vi "Make All Characters Displayable.vi"(11 "String In":string) -> (3 "Escaped String":string)   [LabVIEW 2015, in "VITAC.lvlib"]
uses:
  VITAC.lvlib
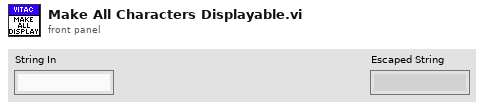
[diagram p1: front panel]
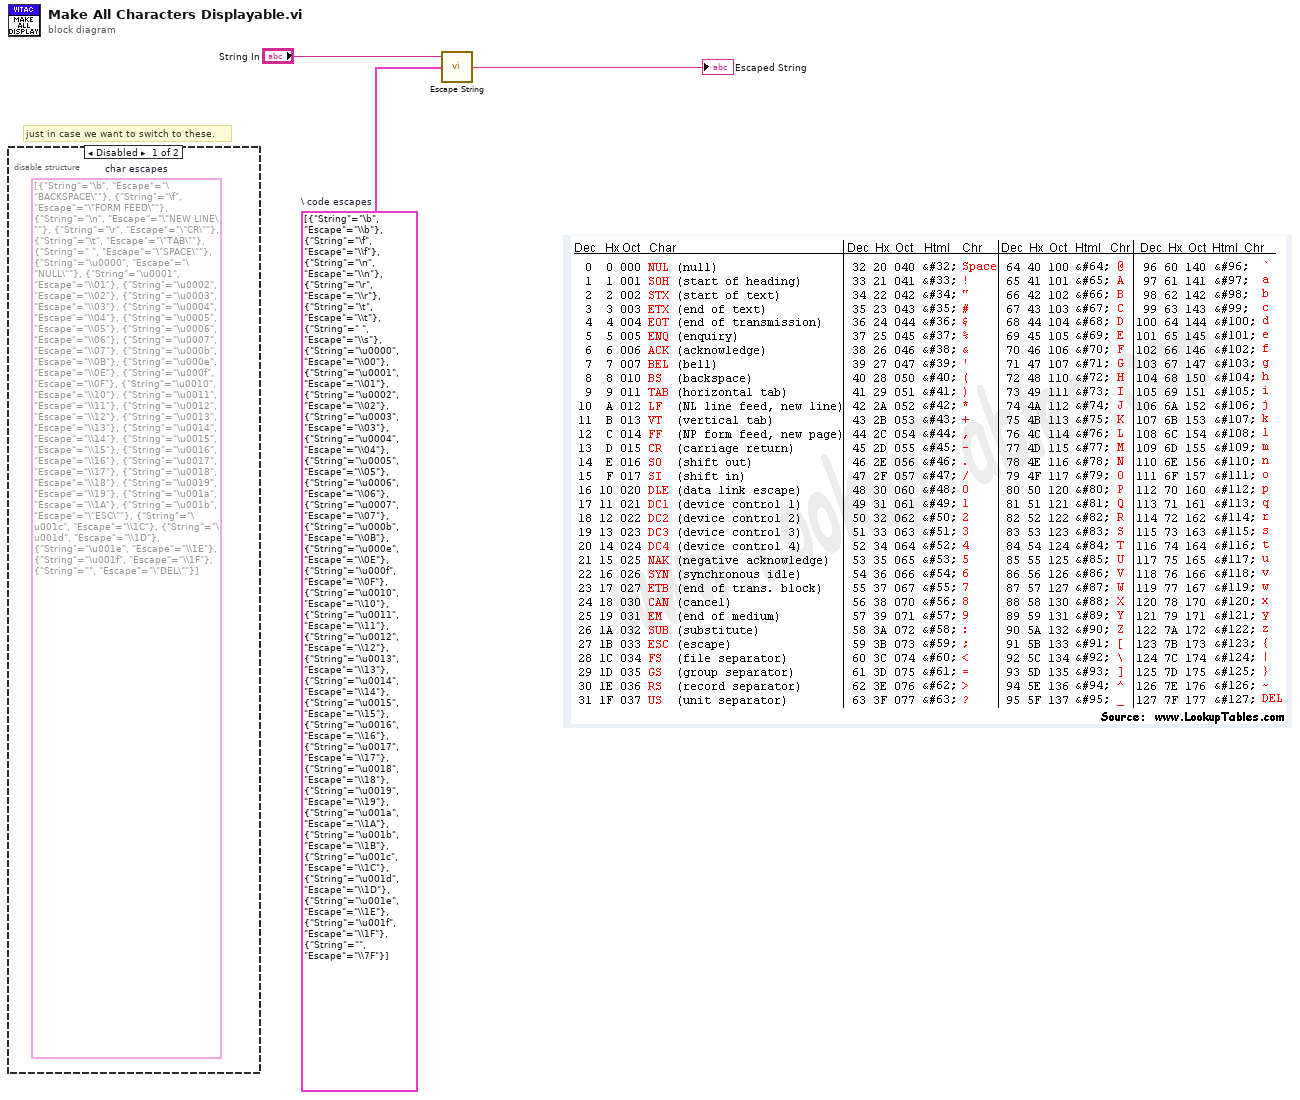
[diagram p0: block diagram]
diagram:
  w3 = cluster{"String":string, "Escape":string}[] [{"String"="\b", "Escape"="\\b"}, {"String"="\f", "Escape"="\\f"}, {"String"="\n", "Escape"="\\n"}, {"String"="\r", "Escape"="\\r"}, {"String"="\t", "Escape"="\\t"}, {"String"=" ", "Escape"="\\s"}, {"String"="\u0000", "Escape"="\\00"}, {"String"="\u0001", "Escape"="\\01"}, {"String"="\u0002", "Escape"="\\02"}, {"String"="\u0003", "Escape"="\\03"}, {"String"="\u0004", "Escape"="\\04"}, {"String"="\u0005", "Escape"="\\05"}, {"String"="\u0006", "Escape"="\\06"}, {"String"="\u0007", "Escape"="\\07"}, {"String"="\u000b", "Escape"="\\0B"}, {"String"="\u000e", "Escape"="\\0E"}, {"String"="\u000f", "Escape"="\\0F"}, {"String"="\u0010", "Escape"="\\10"}, {"String"="\u0011", "Escape"="\\11"}, {"String"="\u0012", "Escape"="\\12"}, {"String"="\u0013", "Escape"="\\13"}, {"String"="\u0014", "Escape"="\\14"}, {"String"="\u0015", "Escape"="\\15"}, {"String"="\u0016", "Escape"="\\16"}, {"String"="\u0017", "Escape"="\\17"}, {"String"="\u0018", "Escape"="\\18"}, {"String"="\u0019", "Escape"="\\19"}, {"String"="\u001a", "Escape"="\\1A"}, {"String"="\u001b", "Escape"="\\1B"}, {"String"="\u001c", "Escape"="\\1C"}, {"String"="\u001d", "Escape"="\\1D"}, {"String"="\u001e", "Escape"="\\1E"}, {"String"="\u001f", "Escape"="\\1F"}, {"String"="", "Escape"="\\7F"}]  # \ code escapes
  # "just in case we want to switch to these."
  n1 = disable-structure shown="Disabled" {
    frame Disabled {
      (unwired) cluster{"String":string, "Escape":string}[] [{"String"="\b", "Escape"="\"BACKSPACE\""}, {"String"="\f", "Escape"="\"FORM FEED\""}, {"String"="\n", "Escape"="\"NEW LINE\""}, {"String"="\r", "Escape"="\"CR\""}, {"String"="\t", "Escape"="\"TAB\""}, {"String"=" ", "Escape"="\"SPACE\""}, {"String"="\u0000", "Escape"="\"NULL\""}, {"String"="\u0001", "Escape"="\\01"}, {"String"="\u0002", "Escape"="\\02"}, {"String"="\u0003", "Escape"="\\03"}, {"String"="\u0004", "Escape"="\\04"}, {"String"="\u0005", "Escape"="\\05"}, {"String"="\u0006", "Escape"="\\06"}, {"String"="\u0007", "Escape"="\\07"}, {"String"="\u000b", "Escape"="\\0B"}, {"String"="\u000e", "Escape"="\\0E"}, {"String"="\u000f", "Escape"="\\0F"}, {"String"="\u0010", "Escape"="\\10"}, {"String"="\u0011", "Escape"="\\11"}, {"String"="\u0012", "Escape"="\\12"}, {"String"="\u0013", "Escape"="\\13"}, {"String"="\u0014", "Escape"="\\14"}, {"String"="\u0015", "Escape"="\\15"}, {"String"="\u0016", "Escape"="\\16"}, {"String"="\u0017", "Escape"="\\17"}, {"String"="\u0018", "Escape"="\\18"}, {"String"="\u0019", "Escape"="\\19"}, {"String"="\u001a", "Escape"="\\1A"}, {"String"="\u001b", "Escape"="\"ESC\""}, {"String"="\u001c", "Escape"="\\1C"}, {"String"="\u001d", "Escape"="\\1D"}, {"String"="\u001e", "Escape"="\\1E"}, {"String"="\u001f", "Escape"="\\1F"}, {"String"="", "Escape"="\"DEL\""}]  # char escapes
    }
    frame Enabled {
    }
  }
  n2 = call <vilib>:"Escape String.vi"("Escapes"=w3, "String in"="String In") -> ("String out"=→"Escaped String":string)  [unwired: 1 in]
